vi "Test_Obj_Oriented.vi"() -> ()   [LabVIEW 2013]
uses:
  MODBUS/MODBUS parameters type.ctl
  <vilib>/DeviceNet/VIAPI/subVIs/DnetIntfConfig.ctl
  Typedef/Array_of_Comm_mode_and_address_types.ctl
  Typedef/Comm_mode_and_address_type.ctl
  Typedef/Comm_mode_type_combo.ctl
  Profibus/Profibus VISA Driver/DF PROFI II.llb/CS_PB_DPV1_MSAC2_InitiateReqData.ctl
  OPC Tester/Controls/OPC Data Output.ctl
  MASTER_OPC.ctl
  Typedef/event var.ctl
  Typedef/Comm ui action type.ctl
  Typedef/Comm_State_enum.ctl
  Typedef/state var.ctl
  OPC Tester/Controls/All Rows Control.ctl
  OPC Tester/Controls/Request Array.ctl
  Typedef/comm_variable_definition.ctl
  OPC Tester/Controls/OPC State.ctl
  Protocol Class/Protocol.lvclass
  MODBUS/MODBUS Class/MODBUS.lvclass
  DeviceNET/DeviceNET Class/DeviceNET.lvclass
  HART/HART Class/HART.lvclass
  Profibus/Profibus Class/Profibus.lvclass
  Typedef/Protocol_enum_type.ctl
  <vilib>/DeviceNet/DeviceNetLIB.lvlib
panel:
  out "Protocol definition":T1(array[cluster]) {"Input" items=["1", "2"]; "Variables" items=["Undefined", "Density", "Delta to", "DZDT DeltaT", "Drive mA", "Board Temp", "Mass Flow", "Tube Frequency", "LPO Amp (Filt)", "RPO Amp (Filt)", "LPO Amp (Pk Det)", "RPO Amp (Pk Det)", "Mass Total", "CP Input Volts", "Temp Line", "Drive Gain%", "Flow cal factor", "Status Word 1", "Status Word 2", "Status Word 3", "Status Word 4", "Status Word 5", "Status Word 6"]}
  out "Data Output":T2 {"Data Out Array"."Cluster.Mode" items=["Modbus-1", "3"]}
  in  "stop":bool
  in  "Profibus ResourceName":refnum<visa-resource-name>="PXI5::11::INSTR"
  in  "Profibus Initiate data":T4={"Communication ref.:"=1, "Send timeout:"=0, "Feat. supp. 1:"=1, "Feat. supp. 2:"=0, "Profile feat. supp. 1:"=0, "Profile feat. supp. 2:"=0, "Profile ID number:"=0, "Addional address parameter"={"S-Type"=FALSE, "S-Length:"=2, "D-Type"=FALSE, "D-Length:"=2, "Data:"=[0, 0, 0, 0]}} {"Addional address parameter"."D-Length:" format="%0.0f"; "Addional address parameter"."S-Length:" format="%0.0f"; "Addional address parameter"."Data:" format="%.0x"; "Feat. supp. 2:" format="%.0x"; "Feat. supp. 1:" format="%.0x"; "Profile feat. supp. 2:" format="%.0x"; "Profile feat. supp. 1:" format="%.0x"; "Profile ID number:" format="%.0x"; "Send timeout:" format="%0.0f"; "Communication ref.:" min=1 max=49 format="%0.0f"}
  in  "Profibus Baud rate":i32(listbox)=6
  in  "Protocol selection\n(appended)":T5 {"Mode" items=["None", "MODBUS", "HART", "Profibus DP", "Profibus PA", "Fieldbus", "DeviceNET"]}
  in  "HART resource name":refnum<visa-resource-name>="HART"
  in  "DeviceNet Interface Configuration":T7={"interface MAC ID"=0, "baud rate"=enum."500000", "poll mode"=enum."Automatic"} {"interface MAC ID" max=63 step=1}
  in  "Interface Name":T8(ring)
  in  "MODBUS resource name":refnum<visa-resource-name>="485"
  in  "MODBUS Serial Parameters":T9={"Mode"=enum."RTU", "Default Slave Address"=111, "MODBUS timeout"=1000, "Baud Rate"=38400, "Parity"=0, "Flow Control"=0} {"Flow Control" items=["None", "XON/XOFF", "RTS/CTS", "XON/XOFF & RTS/CTS", "DTR/DSR", "XON/XOFF & DTR/DSR"]; "Parity" items=["None", "Odd", "Even", "Mark", "Space"]}
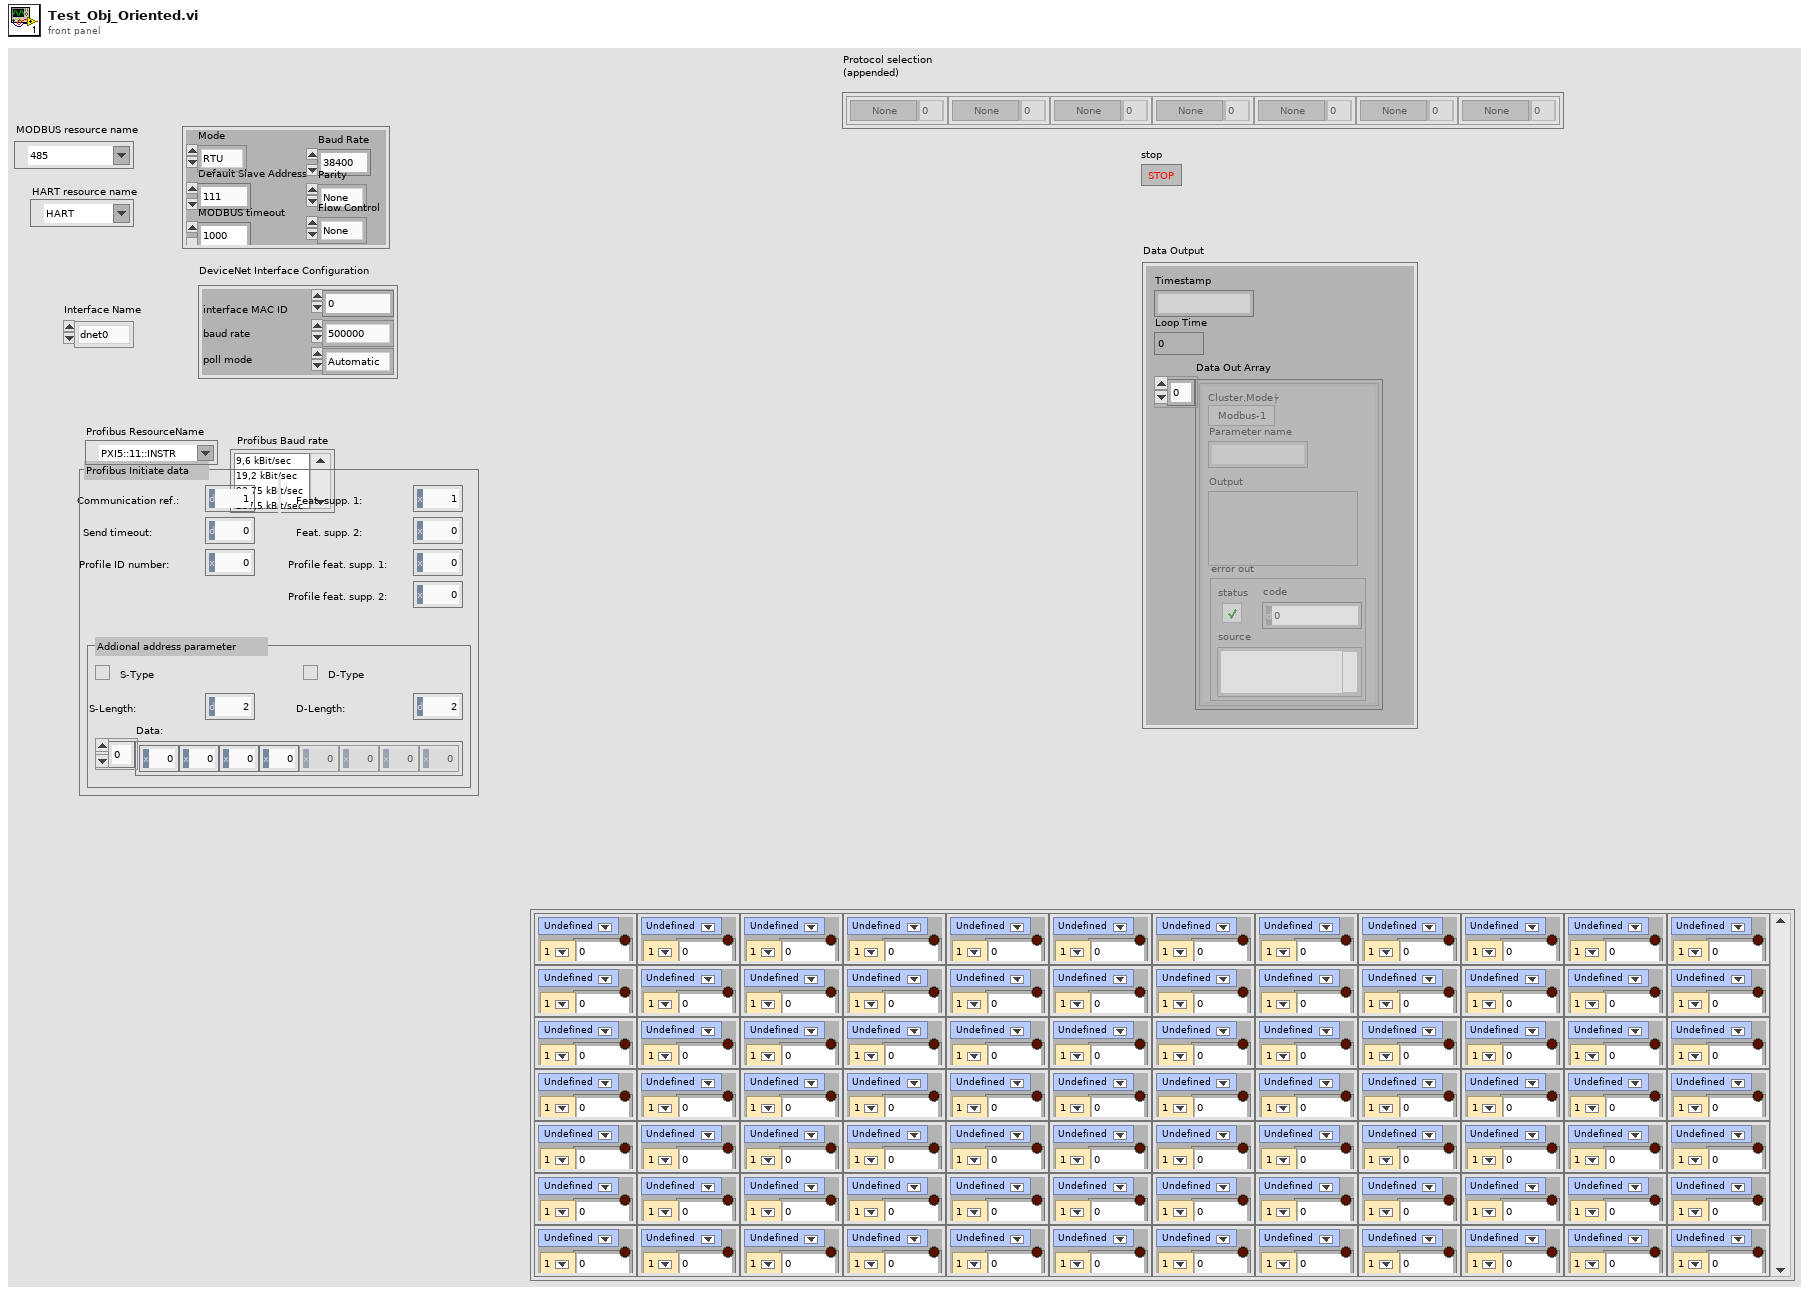
[diagram p1: front panel]
types:
  T1 = cluster{"Variables":u16, "Value":dbl, "Error":bool, "Input":u16, "time stamp":timestamp, "Protocol name":string}[][]
  T2 = typedef "OPC Data Output.ctl" = cluster{"Data Out Array":cluster{"error out":errorcluster, "Output":variant, "Cluster.Mode":T3, "Parameter name":string}[], "Timestamp":string, "Loop Time":dbl}
  T3 = typedef "Comm_mode_type_combo.ctl" = u16
  T4 = typedef "CS_PB_DPV1_MSAC2_InitiateReqData.ctl" = cluster{"Communication ref.:":u8, "Send timeout:":u16, "Feat. supp. 1:":u8, "Feat. supp. 2:":u8, "Profile feat. supp. 1:":u8, "Profile feat. supp. 2:":u8, "Profile ID number:":u16, "Addional address parameter":cluster{"S-Type":bool, "S-Length:":u8, "D-Type":bool, "D-Length:":u8, "Data:":u8[]}}
  T5 = typedef "Array_of_Comm_mode_and_address_types.ctl" = T6[]
  T6 = typedef "Comm_mode_and_address_type.ctl" = cluster{"address":i32, "Mode":T3}
  T7 = typedef "DeviceNetLIB.lvlib/DnetIntfConfig.ctl" = cluster{"interface MAC ID":u32, "baud rate":enum32{"125000", "250000", "500000"}, "poll mode":enum32{"Automatic", "Scanned", "Individual"}}
  T8 = enum16{"dnet0", "dnet1", "dnet2", "dnet3", "dnet4", "dnet5", "dnet6", "dnet7", "dnet8", "dnet9", "dnet10", "dnet11", "dnet12", "dnet13", "dnet14", "dnet15", "dnet16", "dnet17", "dnet18", "dnet19", "dnet20", "dnet21", "dnet22", "dnet23", "dnet24", "dnet25", "dnet26", "dnet27", "dnet28", "dnet29", "dnet30", "dnet31"}
  T9 = typedef "MODBUS parameters type.ctl" = cluster{"Mode":enum16{"RTU", "ASCII"}, "Default Slave Address":u8, "MODBUS timeout":u32, "Baud Rate":u32, "Parity":u16, "Flow Control":u16}
  T10 = typedef "OPC State.ctl" = enum16{"Add New Request", "Run", "Shutdown"}
  T11 = typedef "Request Array.ctl" = T12[]
  T12 = typedef "comm_variable_definition.ctl" = cluster{"General Parameter name":string, "MODBUS Register":i32, "Profibus":cluster{"Friendly name":string, "PA":cluster{"Slot":i32, "Index":i32}, "DP":cluster{"Slot":i32, "Index":i32}, "Tag":string}, "Fieldbus":cluster{"Parameter name":string, "Fieldbus Block":string, "Fieldbus Tag":string}, "data type":enum16{"float", "UINT", "UINT32", "STRING"}, "DeviceNET":cluster{"ClassId":u16, "InstanceId":u16, "AttributeId":u8}, "Cluster":T6, "Length":i32}
  T13 = typedef "All Rows Control.ctl" = string[][]
  T14 = typedef "MASTER_OPC.ctl" = cluster{"Main event var":refnum<user-event>, "VIRef":refnum<vi>, "Data path":path, "Reads":i32, "total number of UUT":i32, "FF refnum":cluster{"Handle1":u32, "Handle2":u32}, "FF device id list":string[], "MODBUS resource name":refnum<visa-resource-name>, "MODBUS Serial Parameters":cluster{"Mode":enum16{"RTU", "ASCII"}, "Default Slave Address":u8, "MODBUS timeout":u32, "Baud Rate":u32, "Parity":u16, "Flow Control":u16}, "Profibus resource name":refnum<visa-resource-name>, "Profibus Communication ref.:":u8, "HART resource name":refnum<visa-resource-name>, "HART long addresses (array)":u8[][], "Comm relay session":refnum<k15>, "Comm UI event":refnum<user-event>, "Write Interval (s)":dbl, "DMM_QUEUE":refnum<queue>, "POWER_QUEUE":refnum<queue>, "\nTHERM_QUEUE":refnum<queue>, "\nCOMM_QUEUE":refnum<queue>, "TIMING_QUEUE":refnum<queue>, "MAIN_QUEUE":refnum<queue>, "Log path":path}
  T15 = typedef "Protocol_enum_type.ctl" = enum16{"None", "MODBUS", "HART", "Fieldbus", "Profibus DP", "Profibus PA", "DeviceNET", "USB"}
  T16 = cluster{"error out":errorcluster, "Output":variant, "Cluster.Mode":T3, "Parameter name":string}
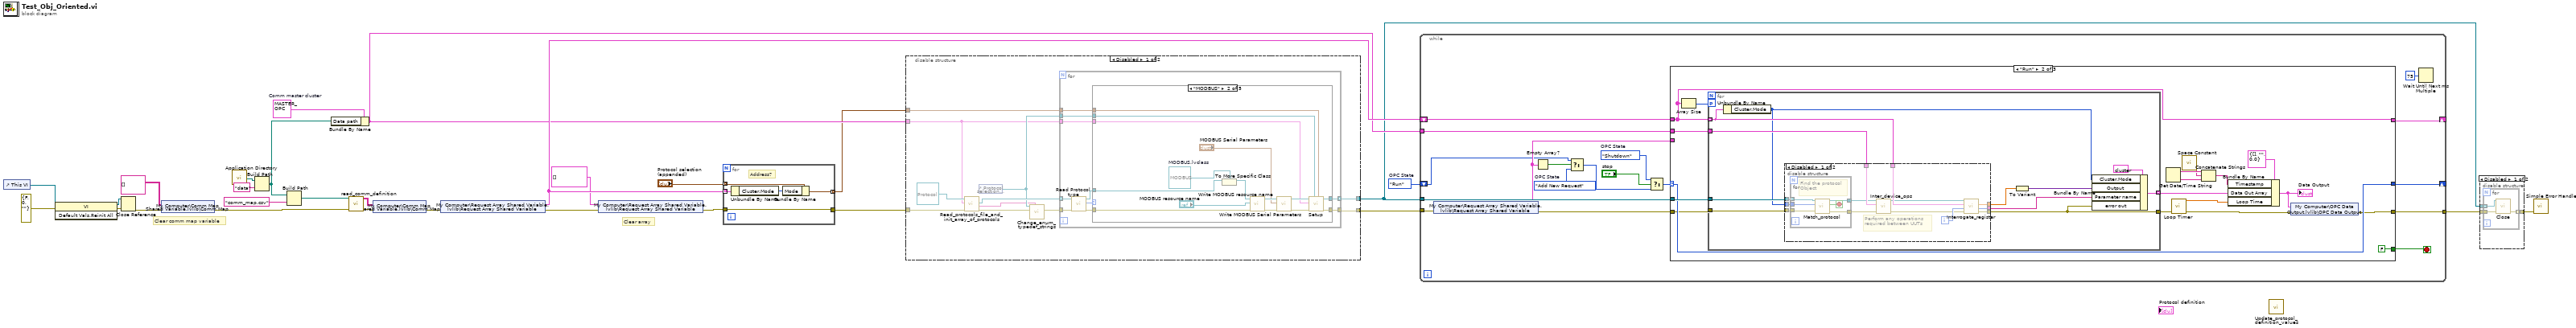
[diagram p0: block diagram]
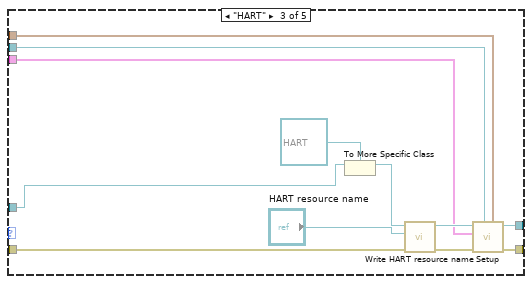
[diagram p4: hidden frame]
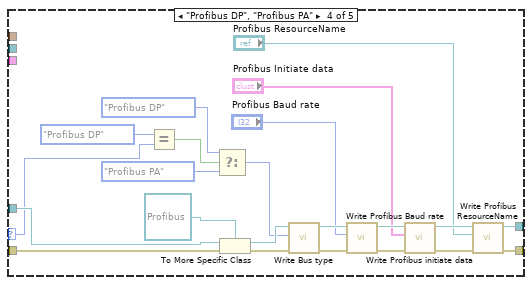
[diagram p5: hidden frame]
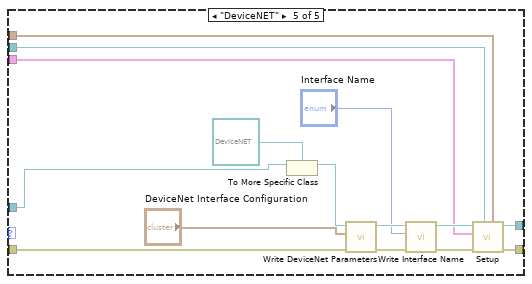
[diagram p6: hidden frame]
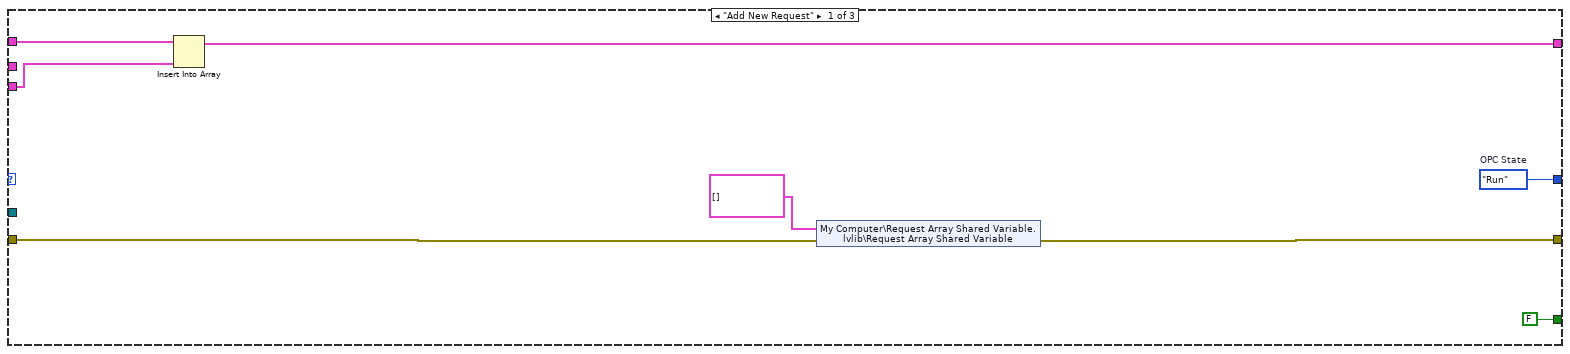
[diagram p8: hidden frame]
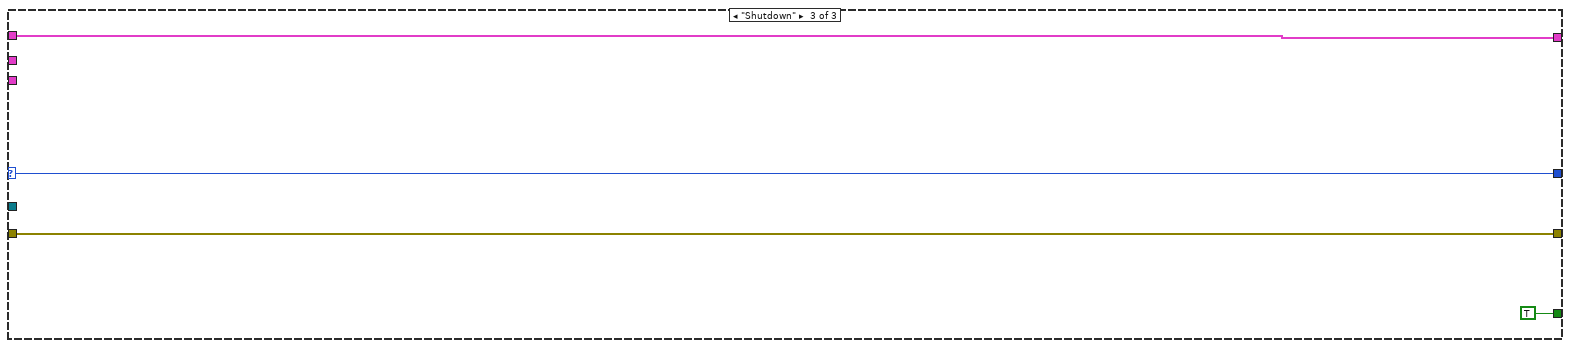
[diagram p10: hidden frame]
diagram:
  w10 = OPC_State."Run"  # OPC State
  w28 = T14 {"Main event var"=refnum, "VIRef"=refnum, "Data path"=path "", "Reads"=0, "total number of UUT"=0, "FF refnum"={"Handle1"=0, "Handle2"=0}, "FF device id list"=[], "MODBUS resource name"="", "MODBUS Serial Parameters"={"Mode"=enum."RTU", "Default Slave Address"=0, "MODBUS timeout"=0, "Baud Rate"=0, "Parity"=0, "Flow Control"=0}, "Profibus resource name"="", "Profibus Communication ref.:"=0, "HART resource name"="", "HART long addresses (array)"=[], "Comm relay session"="", "Comm UI event"=refnum, "Write Interval (s)"=5.0, "DMM_QUEUE"=refnum, "POWER_QUEUE"=refnum, "\nTHERM_QUEUE"=refnum, "\nCOMM_QUEUE"=refnum, "TIMING_QUEUE"=refnum, "MAIN_QUEUE"=refnum, "Log path"=path ""}  # Comm master cluster
  # "Clear array"
  # "Clear comm map variable"
  n1 = control-ref of="This VI"() -> (w18:refnum<vi>)
  n2 = invoke class="VI" method="Default Vals.Reinit All"(reference=w18, error in=errorcluster {"status"=FALSE, "code"=0, "source"=""} ("error constant")) -> (reference out=w21:refnum<vi>, error out=w20:errorcluster)  [unwired: 1 in, 1 out]
  n3 = Close Reference(reference=w21, error in (no error)=w20) -> (error out=w17:errorcluster)
  n4 = shared-variable "My Computer\\Comm Map Shared Variable.lvlib\\Comm Map"(T13 [] ("Comm Map"), error in=w17) -> (error out=w1:errorcluster)
  n5 = call <vilib>:"Application Directory.vi"() -> ("Application Directory"=w6:path)
  n6 = Build Path(base path=w6, name or relative path="data") -> (appended path=w2:path)
  n7 = Build Path(base path=w2, name or relative path="comm_map.csv") -> (appended path=w4:path)
  n8 = Bundle By Name(cluster=w28, "Data path"=w2) -> (w25:T14)
  n9 = call "read_comm_definition.vi"("error in (no error)"=w1, "file path (dialog if empty)"=w4) -> ("error out"=w23:errorcluster, "all rows"=w24:string[][])  [unwired: 7 in, 1 out]
  n10 = shared-variable "My Computer\\Comm Map Shared Variable.lvlib\\Comm Map"(w24, error in=w23) -> (error out=w22:errorcluster)
  n11 = shared-variable "My Computer\\Request Array Shared Variable.lvlib\\Request Array Shared Variable"(error in=w22) -> (w29:T11, error out=w13:errorcluster)
  n12 = shared-variable "My Computer\\Request Array Shared Variable.lvlib\\Request Array Shared Variable"(T11 [] ("Request Array Shared Variable"), error in=w13) -> (error out=w12:errorcluster)
  n13 = for {
    tunnel: "Protocol selection\n(appended)" -> [w34] mode=indexing
    tunnel: w29 -> [w33] mode=indexing
    tunnel: w12 -> [w30]
    tunnel: [w31] -> w8 mode=indexing
    tunnel: [w30] -> w15
    # "Address?"
    n14 = Unbundle By Name(w33) -> ("Cluster.Mode"=w32:T3)
    n15 = Bundle By Name(cluster=w34, "Mode"=w32) -> (w31:T6)
  }
  n16 = disable-structure shown="Disabled" {
    disable-tunnel: [w43 _] -> w27
    disable-tunnel: w25 -> [w38 _]
    disable-tunnel: w8 -> [w37 _]
    disable-tunnel: w15 -> [w36 _]
    disable-tunnel: [w35 _] -> w14
    frame Disabled {
      n17 = call-dynamic "Read_protocols_file_and_init_array_of_protocols.vi"("error in (no error)"=w36, "Comm master cluster"=w38, "Protocol in"=refnum<class "Protocol.lvclass"> refnum) -> ("error out"=w40:errorcluster, "Array of configured protocols"=w41:string[], "Array of Protocols out"=w44:refnum<class "Protocol.lvclass">[])  [unwired: 5 in, 1 out]
      n18 = control-ref of="Protocol selection\n(appended)"() -> (w42:refnum<vi>)
      n19 = call "Change_enum_typedef_strings.vi"("Strings []"=w41, "error in (no error)"=w40, "protocol selection ref"=w42) -> ("error out"=w39:errorcluster)  [unwired: 8 in]
      n20 = for {
        tunnel: w44 -> [w55] mode=indexing
        tunnel: [w52] -> w35 mode=indexing
        tunnel: [w51] -> w43
        tunnel: w38 -> [w49]
        tunnel: w37 -> [w48]
        tunnel: w42 -> [w47]
        tunnel: w39 -> [w46]
        n21 = call-dynamic "Read Protocol type.vi"("error in (no error)"=w46, "Protocol in"=w55) -> ("error out"=w50:errorcluster, "Protocols"=w54:T15, "Protocol out"=w53:refnum<class "Protocol.lvclass">)  [unwired: 7 in]
        n22 = case shown="\"MODBUS\"" w54 {
          selector: w54 -> [_ _ _ w93 _]
          tunnel: w53 -> [w57 w72 w84 w105 w121]
          tunnel: [w57 w70 w79 w85 w120] -> w52
          tunnel: [w56 w62 w76 w101 w119] -> w51
          tunnel: w50 -> [w56 w61 w81 w95 w113]
          tunnel: w49 -> [_ w60 w78 _ w109]
          tunnel: w48 -> [_ w59 w75 _ w107]
          tunnel: w47 -> [_ w58 w74 _ w108]
          frame "None", Default {
          }
          frame "MODBUS" {
            w71 = refnum<class "MODBUS.lvclass"> refnum  # MODBUS.lvclass
            n23 = To More Specific Class(target class=w71, reference=w72) -> (specific class reference=w69:refnum<class "MODBUS.lvclass">)  [unwired: 1 in, 1 out]
            n24 = call-dynamic "Write MODBUS resource name.vi"("error in (no error)"=w61, "MODBUS resource name"="MODBUS resource name", "MODBUS in"=w69) -> ("error out"=w67:errorcluster, "MODBUS out"=w66:refnum<class "MODBUS.lvclass">)  [unwired: 7 in]
            n25 = call-dynamic "Write MODBUS Serial Parameters.vi"("error in (no error)"=w67, "MODBUS Serial Parameters"="MODBUS Serial Parameters", "MODBUS in"=w66) -> ("error out"=w63:errorcluster, "MODBUS out"=w64:refnum<class "MODBUS.lvclass">)  [unwired: 7 in]
            n26 = call-dynamic "Setup.vi"("Protocol selection\n(appended)"=w59, "protocol selection ref"=w58, "error in (no error)"=w63, "Comm master cluster in"=w60, "MODBUS in"=w64) -> ("error out"=w62:errorcluster, "MODBUS out"=w70:refnum<class "MODBUS.lvclass">)  [unwired: 5 in]
          }
          frame "HART" {
            n27 = To More Specific Class(target class=refnum<class "HART.lvclass"> refnum ("HART.lvclass"), reference=w84) -> (specific class reference=w83:refnum<class "HART.lvclass">)  [unwired: 1 in, 1 out]
            n28 = call-dynamic "Write HART resource name.vi"("error in (no error)"=w81, "HART resource name"="HART resource name", "HART in"=w83) -> ("error out"=w77:errorcluster, "HART out"=w80:refnum<class "HART.lvclass">)  [unwired: 7 in]
            n29 = call-dynamic "Setup.vi"("Protocol selection\n(appended)"=w75, "protocol selection ref"=w74, "error in (no error)"=w77, "Comm master cluster in"=w78, "HART in"=w80) -> ("error out"=w76:errorcluster, "HART out"=w79:refnum<class "HART.lvclass">)  [unwired: 5 in]
          }
          frame "Profibus DP", "Profibus PA" {
            n30 = Equal?(x=Protocol_enum_type."Profibus DP" ("Protocols"), y=w93) -> (x = y?=w92:bool)
            n31 = Select(t=enum16{"Profibus DP", "Profibus PA"}."Profibus DP" ("Bus type"), s=w92, f=enum16{"Profibus DP", "Profibus PA"}."Profibus PA" ("Bus type")) -> (s? t:f=w89:enum16{"Profibus DP", "Profibus PA"})
            n32 = To More Specific Class(target class=refnum<class "Profibus.lvclass"> refnum ("Profibus.lvclass"), reference=w105, error in=w95) -> (specific class reference=w97:refnum<class "Profibus.lvclass">, error out=w96:errorcluster)
            n33 = call-dynamic "Write Bus type.vi"("error in (no error)"=w96, "Bus type"=w89, "Profibus in"=w97) -> ("error out"=w104:errorcluster, "Profibus out"=w100:refnum<class "Profibus.lvclass">)  [unwired: 7 in]
            n34 = call-dynamic "Write Profibus Baud rate.vi"("error in (no error)"=w104, "Profibus Baud rate"="Profibus Baud rate", "Profibus in"=w100) -> ("error out"=w103:errorcluster, "Profibus out"=w99:refnum<class "Profibus.lvclass">)  [unwired: 7 in]
            n35 = call-dynamic "Write Profibus initiate data.vi"("error in (no error)"=w103, "Initiate data"="Profibus Initiate data", "Profibus in"=w99) -> ("error out"=w102:errorcluster, "Profibus out"=w98:refnum<class "Profibus.lvclass">)  [unwired: 7 in]
            n36 = call-dynamic "Write Profibus ResourceName.vi"("error in (no error)"=w102, "Profibus ResourceName"="Profibus ResourceName", "Profibus in"=w98) -> ("error out"=w101:errorcluster, "Profibus out"=w85:refnum<class "Profibus.lvclass">)  [unwired: 7 in]
          }
          frame "DeviceNET" {
            n37 = To More Specific Class(target class=refnum<class "DeviceNET.lvclass"> refnum ("DeviceNET.lvclass"), reference=w121) -> (specific class reference=w110:refnum<class "DeviceNET.lvclass">)  [unwired: 1 in, 1 out]
            n38 = call-dynamic "Write DeviceNet Parameters.vi"("error in (no error)"=w113, "DeviceNet Interface Configuration"="DeviceNet Interface Configuration", "DeviceNET in"=w110) -> ("error out"=w112:errorcluster, "DeviceNET out"=w117:refnum<class "DeviceNET.lvclass">)  [unwired: 7 in]
            n39 = call-dynamic "Write Interface Name.vi"("error in (no error)"=w112, "Interface Name"="Interface Name", "DeviceNET in"=w117) -> ("error out"=w111:errorcluster, "DeviceNET out"=w116:refnum<class "DeviceNET.lvclass">)  [unwired: 7 in]
            n40 = call-dynamic "Setup.vi"("Protocol selection\n(appended)"=w107, "protocol selection ref"=w108, "error in (no error)"=w111, "Comm master cluster in"=w109, "DeviceNET in"=w116) -> ("error out"=w119:errorcluster, "DeviceNET out"=w120:refnum<class "DeviceNET.lvclass">)  [unwired: 5 in]
          }
        }
      }
    }
    frame Enabled {
    }
  }
  n41 = while {
    tunnel: w14 -> [w139]
    tunnel: w27 -> [w131]
    tunnel: [w136] -> w26
    tunnel: w25 -> [w138]
    shift-right: [w124] -> _
    shift-left: w29 -> [w137]
    shift-right: [w122] -> _
    shift-left: w10 -> [w125]
    stop <- w123 stop-if-true
    w128 = OPC_State."Add New Request"  # OPC State
    w132 = OPC_State."Shutdown"  # OPC State
    n42 = shared-variable "My Computer\\Request Array Shared Variable.lvlib\\Request Array Shared Variable"(error in=w131) -> (w126:T11, error out=w130:errorcluster)
    n43 = Empty Array?(array=w126) -> (empty?=w129:bool)
    n44 = Select(t=w125, s=w129, f=w128) -> (s? t:f=w127:T10)
    n45 = Select(t=w132, s="stop", f=w127) -> (s? t:f=w134:T10)
    n46 = case shown="\"Run\"" w134 {
      selector: w134 -> [_ w160 w199]
      tunnel: w139 -> [_ w165 _]
      tunnel: w138 -> [_ w164 _]
      tunnel: w130 -> [w144 w159 w197]
      tunnel: w137 -> [w147 w161 w200]
      tunnel: [w143 w150 w197] -> w136
      tunnel: w126 -> [w146 _ _]
      tunnel: [w145 w161 w200] -> w124
      tunnel: [FALSE FALSE TRUE] -> w123
      tunnel: [w140 w160 w199] -> w122
      frame "Add New Request" {
        w140 = OPC_State."Run"  # OPC State
        n47 = Insert Into Array(array=w147, new element=w146) -> (w145:T11)  [unwired: 1 in]
        n48 = shared-variable "My Computer\\Request Array Shared Variable.lvlib\\Request Array Shared Variable"(T11 [] ("Request Array Shared Variable"), error in=w144) -> (error out=w143:errorcluster)
      }
      frame "Run" {
        n49 = Array Size(array=w161) -> (size(s)=w163:i32)
        n50 = for {
          tunnel: w165 -> [w176]
          tunnel: [w172] -> w155
          tunnel: w161 -> [w173] mode=indexing
          tunnel: w164 -> [w175]
          tunnel: w159 -> [w174]
          workers-P: w163 -> [_]
          tunnel: [w171] -> w153 mode=indexing
          i -> [w177]
          n51 = Unbundle By Name(w173) -> ("Cluster.Mode"=w168:T3)
          n52 = disable-structure shown="Disabled" {
            disable-tunnel: w177 -> [w190 _]
            disable-tunnel: w176 -> [w189 _]
            disable-tunnel: w175 -> [w188 _]
            disable-tunnel: w174 -> [w187 _]
            disable-tunnel: w173 -> [w186 _]
            disable-tunnel: [w185 _] -> w172
            disable-tunnel: [w184 _] -> w170
            disable-tunnel: w168 -> [w179 _]
            disable-tunnel: [w178 _] -> w166
            frame Disabled {
              # "Perform any operations \nrequired between UUTs"
              n53 = for {
                tunnel: w189 -> [w196] mode=indexing
                tunnel: w179 -> [w195]
                tunnel: [w193] -> w183
                tunnel: [w192] -> w182
                tunnel: w187 -> [w191]
                stop <- w194 stop-if-true
                # "Find the protocol\nObject"
                n54 = call-dynamic "Match_protocol.vi"("error in (no error)"=w191, "Protocol type"=w195, "Protocol in"=w196) -> ("error out"=w192:errorcluster, "Match"=w194:bool, "Protocol out"=w193:refnum<class "Protocol.lvclass">)  [unwired: 6 in]
              }
              n55 = call-dynamic "Inter_device_ops.vi"("error in (no error)"=w182, "Comm master cluster in"=w188, "Protocol in"=w183) -> ("error out"=w180:errorcluster, "Protocol out"=w181:refnum<class "Protocol.lvclass">)  [unwired: 7 in]
              n56 = call-dynamic "Interrogate_register.vi"("error in (no error)"=w180, "UUT Index"=w190, "Register mutli-protocol location"=w186, "Protocol in"=w181) -> ("error out"=w185:errorcluster, "Parameter name"=w178:string, "output"=w184:sgl)  [unwired: 3 in, 2 out]
            }
            frame Enabled {
            }
          }
          n57 = To Variant(anything=w170) -> (Variant=w167:variant)
          n58 = Bundle By Name(cluster=T16 {"error out"={"status"=FALSE, "code"=0, "source"=""}, "Output"=variant, "Cluster.Mode"=0, "Parameter name"=""} ("Data Out"), "Cluster.Mode"=w168, "Output"=w167, "Parameter name"=w166, "error out"=w172) -> (w171:T16)
        }
        n59 = Get Date/Time String() -> (date string=w158:string, time string=w157:string)  [unwired: 3 in]
        n60 = call "Loop Timer.vi"("error in (no error)"=w155) -> ("error out"=w148:errorcluster, "Loop Time"=w152:dbl)  [unwired: 9 in]
        n61 = call <vilib>:"Space Constant.vi"() -> ("String"=w156:string)
        n62 = Concatenate Strings(w158, w156, w157) -> (w151:string)
        n63 = Bundle By Name(cluster=T2 {"Data Out Array"=[], "Timestamp"="", "Loop Time"=0.0} ("Data Output"), "Timestamp"=w151, "Data Out Array"=w153, "Loop Time"=w152) -> (w149:T2)
        "Data Output" <- w149
        n64 = shared-variable "My Computer\\OPC Data Output.lvlib\\OPC Data Output"(w149, error in=w148) -> (error out=w150:errorcluster)
      }
      frame "Shutdown" {
      }
    }
    n65 = Wait Until Next ms Multiple(millisecond multiple=u32 75) -> ()  [unwired: 1 out]
  }
  n66 = call "Update_protocol_definition_values.vi"() -> ()  [unwired: 11 in, 1 out]
  n67 = disable-structure shown="Disabled" {
    disable-tunnel: [w203 _] -> w9
    disable-tunnel: w26 -> [w202 _]
    disable-tunnel: w14 -> [w201 _]
    frame Disabled {
      n68 = for {
        tunnel: w201 -> [w206] mode=indexing
        tunnel: [w205] -> w203 mode=indexing
        tunnel: w202 -> [w204]
        n69 = call-dynamic "Close.vi"("error in (no error)"=w204, "Protocol in"=w206) -> ("error out"=w205:errorcluster)  [unwired: 8 in, 1 out]
      }
    }
    frame Enabled {
    }
  }
  n70 = call <vilib>:"Simple Error Handler.vi"("error in (no error)"=w9) -> ()  [unwired: 4 in, 5 out]
